vi "CRYString terminator definite.vi"(10 "Terminator":string, 11 "String in":string) -> (3 "String out":string)   [LabVIEW 2013]
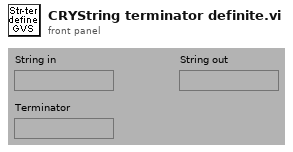
[diagram p1: front panel]
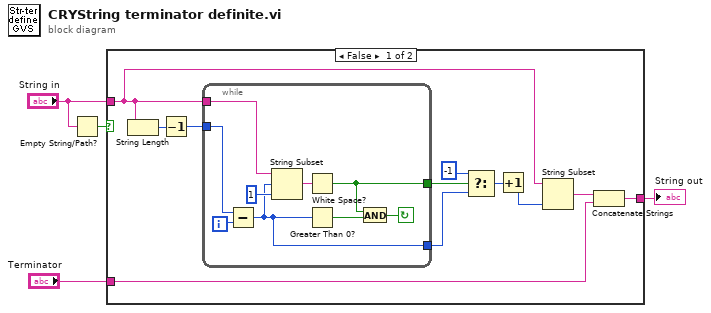
[diagram p0: block diagram]
diagram:
  n1 = Empty String/Path?(string/path="String in") -> (empty?=w2:bool)
  n2 = case shown="False" w2 {
    tunnel: "String in" -> [w10 _]
    tunnel: "Terminator" -> [w7 w25]
    tunnel: [w5 w25] -> w1
    frame False {
      n3 = String Length(string=w10) -> (length=w15:i32)
      n4 = Decrement(x=w15) -> (x-1=w14:i32)
      n5 = while {
        tunnel: [w16] -> w12
        tunnel: [w17] -> w13
        tunnel: w14 -> [w23]
        tunnel: w10 -> [w21]
        i -> [w24]
        stop <- w18 continue-if-true
        n6 = Subtract(x=w23, y=w24) -> (x-y=w16:i32)
        n7 = String Subset(string=w21, offset (0)=w16, length (rest)=1) -> (substring=w20:string)
        n8 = White Space?(1:w20) -> (0:w17:bool)
        n9 = Greater Than 0?(x=w16) -> (x > 0?=w19:bool)
        n10 = And(x=w17, y=w19) -> (x .and. y?=w18:bool)
      }
      n11 = Select(t=-1, s=w13, f=w12) -> (s? t:f=w8:i32)
      n12 = Increment(x=w8) -> (x+1=w9:i32)
      n13 = String Subset(string=w10, length (rest)=w9) -> (substring=w6:string)  [unwired: 1 out]
      n14 = Concatenate Strings(w6, w7) -> (w5:string)
    }
    frame True {
    }
  }
  "String out" <- w1
